vi "createViReference.vi"(8 "error in (no error)":errorcluster, 9 "topic":string, 10 "SAL_Library":string="SALLV_EXA.lvlib:", 11 "ProgrammaticInitialization in":refnum<class "ProgrammaticInitialization.lvclass">) -> (0 "error out":errorcluster, 3 "ProgrammaticInitialization out":refnum<class "ProgrammaticInitialization.lvclass">)   [LabVIEW 2016, in "ProgrammaticInitialization.lvclass"]
uses:
  ProgrammaticInitialization.lvclass
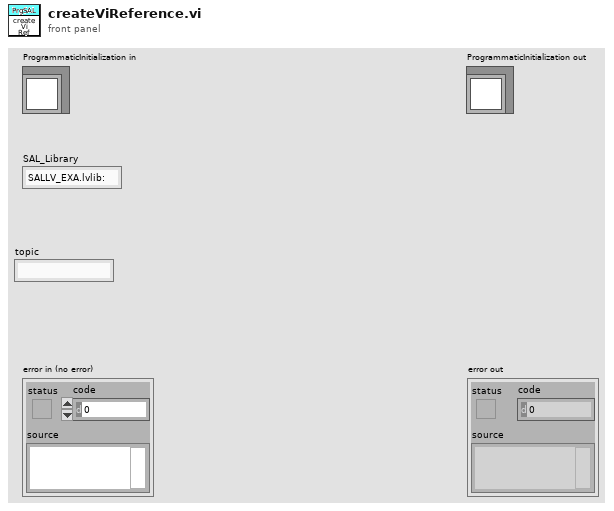
[diagram p1: front panel]
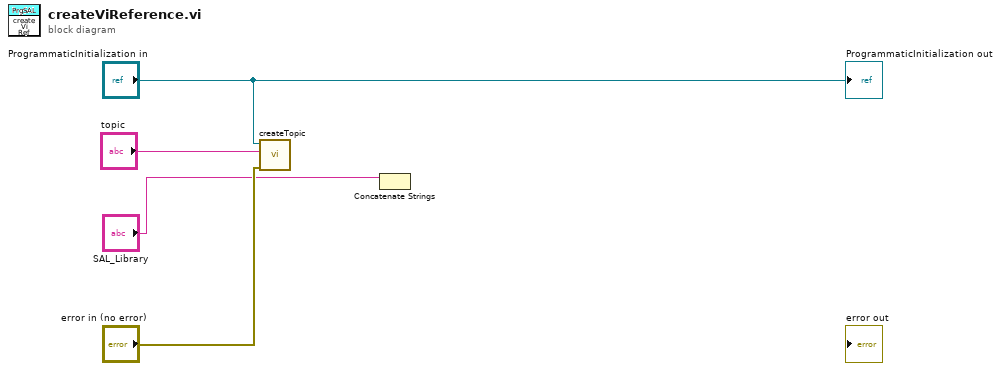
[diagram p0: block diagram]
diagram:
  n1 = call "createTopic.vi"("error in (no error)"="error in (no error)", "topic"="topic", "ProgrammaticInitialization in"="ProgrammaticInitialization in") -> ()  [unwired: 6 in, 3 out]
  n2 = Concatenate Strings("SAL_Library") -> ()  [unwired: 1 in, 1 out]
  "ProgrammaticInitialization out" <- "ProgrammaticInitialization in"
